vi "系统设置全局变量.vi"() -> ()   [LabVIEW 2016]
panel:
  in  "模块启用":T1={"环境动力"=TRUE, "氨氮"=TRUE, "总磷"=TRUE, "总氮"=TRUE, "高锰酸盐指数"=TRUE, "化学需氧量"=FALSE, "多参数"=TRUE, "加标回收"=FALSE, "GPS"=TRUE, "多参数版本"=enum."集成"}
  in  "服务器":T2={"host"="27.154.58.30", "port"=8020, "user"="std", "password"="std23506", "远端地址"="/浮船/浮船V1/浮船水质自动监测系统.exe"}
  in  "站点系列号":string
  in  "站点名称":string
  in  "系统重启设置":T3 {"分" max=59 format="%02.0f"; "时" max=23 format="%02.0f"}
  # "频次："
  # "时间："
  # "："
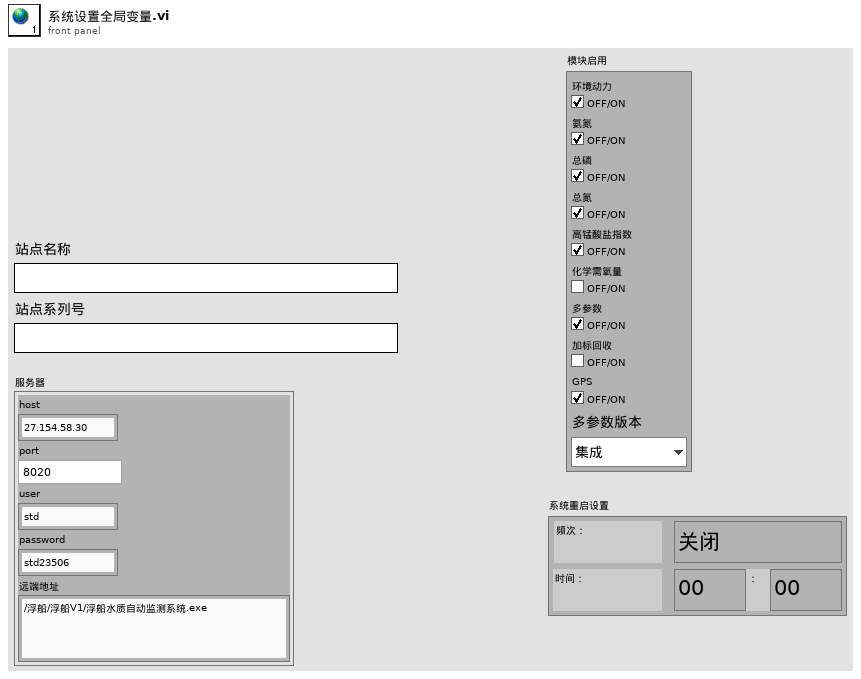
[diagram p1: front panel]
types:
  T1 = cluster{"环境动力":bool, "氨氮":bool, "总磷":bool, "总氮":bool, "高锰酸盐指数":bool, "化学需氧量":bool, "多参数":bool, "加标回收":bool, "GPS":bool, "多参数版本":enum16{"集成", "原位"}}
  T2 = cluster{"host":string, "port":u16, "user":string, "password":string, "远端地址":string}
  T3 = cluster{"频次":enum16{"关闭", "每天", "星期一", "星期二", "星期三", "星期四", "星期五", "星期六", "星期日"}, "时":u16, "分":u16}
diagram:
